vi "Problem1.3-ResetSubVI.vi"(10 "Clust Refnum in":refnum<vi>, 11 "Cluster in":refnum<vi>) -> (0 "error out":errorcluster)   [LabVIEW 2019]
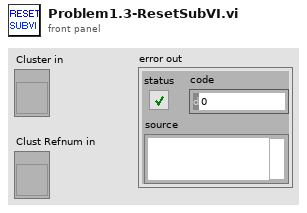
[diagram p1: front panel]
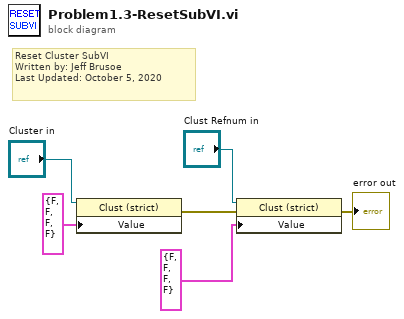
[diagram p0: block diagram]
diagram:
  # "Reset Cluster SubVI\nWritten by: Jeff Brusoe\nLast Updated: October 5, 2020"
  n1 = property on="Property Node" class="Clust (strict)"(reference="Cluster in", "Value"=cluster{"1":bool, "2":bool, "4":bool, "8":bool} {"1"=FALSE, "2"=FALSE, "4"=FALSE, "8"=FALSE} ("Input Cluster")) -> (error out=w5:errorcluster)  [unwired: 1 in, 1 out]
  n2 = property on="Property Node" class="Clust (strict)"(reference="Clust Refnum in", error in=w5, "Value"=cluster{"1":bool, "2":bool, "4":bool, "8":bool} {"1"=FALSE, "2"=FALSE, "4"=FALSE, "8"=FALSE} ("Input Cluster 2")) -> (error out=→"error out":errorcluster)  [unwired: 1 out]
